vi "Start Detailed View.vi"(8 "error in (no error)":errorcluster, 9 "Start Subsystem":string, 10 "Server URL":refnum<k21>, 11 "Client Message Queues":T1) -> (0 "error out":errorcluster, 3 "VI Reference":refnum<vi>)   [LabVIEW 2024]
doc: "Starts the Detailed View."
uses:
  Shared/Message Queue/Client Message Queues.ctl
  Shared/Message Queue/Message Cluster.ctl
  Shared/Message Queue.lvlib
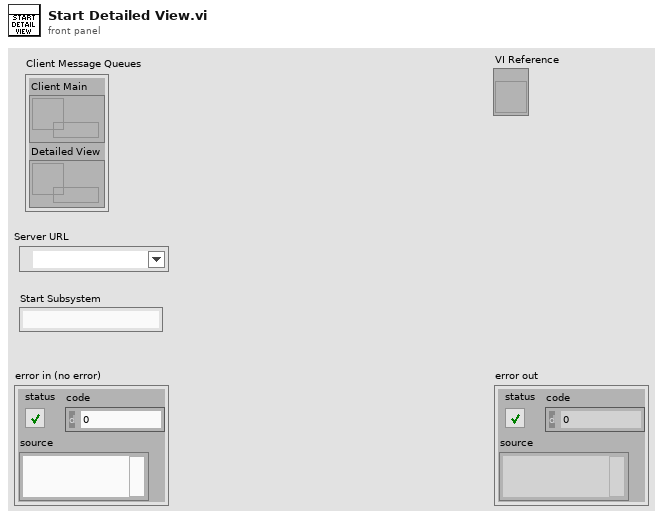
[diagram p1: front panel]
types:
  T1 = typedef "Message Queue.lvlib/Client Message Queues.ctl" = cluster{"Client Main":refnum<queue>, "Detailed View":refnum<queue>}
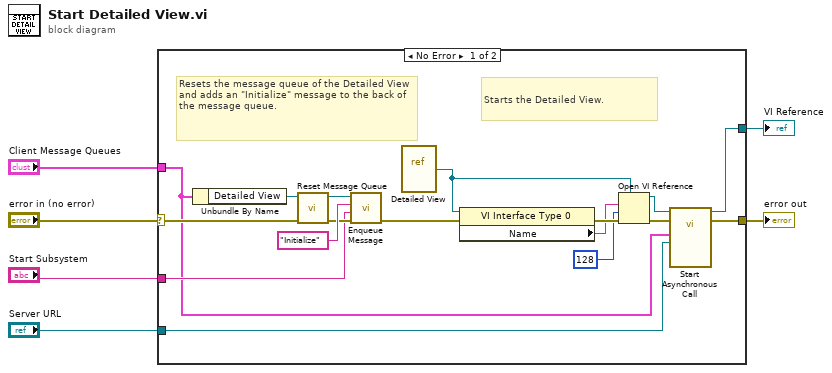
[diagram p0: block diagram]
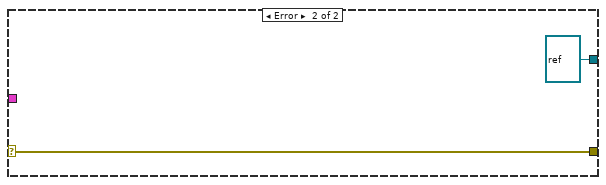
[diagram p2: hidden frame]
diagram:
  n1 = case shown="No Error" "error in (no error)" {
    selector: "error in (no error)" -> [w19 w25]
    tunnel: [w10 w25] -> w5
    tunnel: "Client Message Queues" -> [w7 _]
    tunnel: "Server URL" -> [w8 _]
    tunnel: [w9 refnum<vi> refnum] -> w3
    tunnel: "Start Subsystem" -> [w18 _]
    frame No Error {
      # "Resets the message queue of the Detailed View and adds an \"Initialize\" message to the back of the message queue."
      # "Starts the Detailed View."
      n2 = Unbundle By Name(w7) -> ("Detailed View"=w22:refnum<queue>)
      n3 = call "Reset Message Queue.vi"("error in (no error)"=w19, "Message Queue"=w22) -> ("error out"=w20:errorcluster, "dup Message Queue"=w21:refnum<queue>)  [unwired: 8 in]
      n4 = call "Enqueue Message.vi"("error in (no error)"=w20, "Message Data"=w18, "Message"="Initialize", "Message Queue"=w21) -> ("error out"=w11:errorcluster)  [unwired: 6 in, 1 out]
      n5 = vi-ref "Detailed View.vi"() -> (w12:refnum<vi>)
      n6 = property class="VI Interface Type 0"(reference=w12, error in=w11) -> (error out=w17:errorcluster, "Name"=w14:string)  [unwired: 1 out]
      n7 = Open VI Reference(type specifier VI Refnum (for type only)=w12, vi path=w14, options=128, error in (no error)=w17) -> (vi reference=w13:refnum<vi>, error out=w16:errorcluster)  [unwired: 2 in]
      n8 = call-by-ref "Start Asynchronous Call"(reference=w13, error in=w16, "Server URL"=w8, "Client Message Queues"=w7) -> (reference out=w9:refnum<vi>, error out=w10:errorcluster)  [unwired: 10 in]
    }
    frame Error {
    }
  }
  "error out" <- w5
  "VI Reference" <- w3
